vi "Configure Trigger (Glitch).vi"(0 "VISA resource name":refnum<visa-resource-name>, 1 "Maximum Width (1.5E-9s)":dbl=1.5e-09, 5 "Trigger Source (1: Channel 1)":i32(ring)=1 items=["Channel 1"=1, "Channel 2"=2, "Channel 3"=3, "Channel 4"=4, "Digital 0"=13, "Digital 1"=14, "Digital 2"=15, "Digital 3"=16, "Digital 4"=17, "Digital 5"=18, "Digital 6"=19, "Digital 7"=20, "Digital 8"=21, "Digital 9"=22, "Digital 10"=23, "Digital 11"=24, "Digital 12"=25, "Digital 13"=26, "Digital 14"=27, "Digital 15"=28], 7 "Trigger Level (0.0 V)":dbl, 9 "Trigger Polarity (0: Positive)":i32(ring) items=["Positive", "Negative"], 11 "error in (no error)":errorcluster) -> (4 "VISA resource name out":refnum<visa-resource-name>, 15 "error out":errorcluster)   [LabVIEW 2012, in "Agilent 8000 Series.lvlib"]
doc: "Configures the glitch trigger. A glitch trigger occurs when the trigger signal has a pulse with a width that is less than the glitch width. You specify the glitch width in the Glitch Width parameter. You specify the polarity of the pulse with the Glitch Polarity parameter. The trigger does not actually occur until the edge of a pulse that corresponds to the Glitch Width and Glitch Polarity crosses the threshold you specify in the Trigger Level parameter. \n\n<B>Note:</B>\n80000 series oscilloscopes <B>do not</B> support Digital Channels."
uses:
  Agilent 8000 Series.lvlib
panel:
  # "80000 Series Oscilloscopes\ndo not support digital channels"
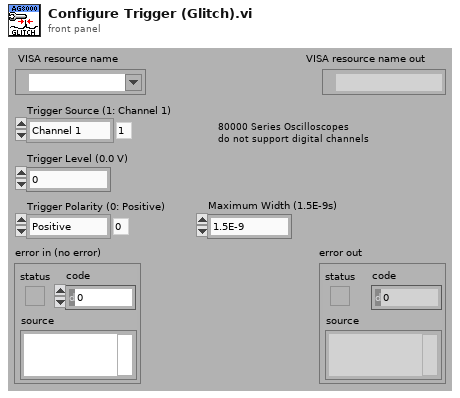
[diagram p1: front panel]
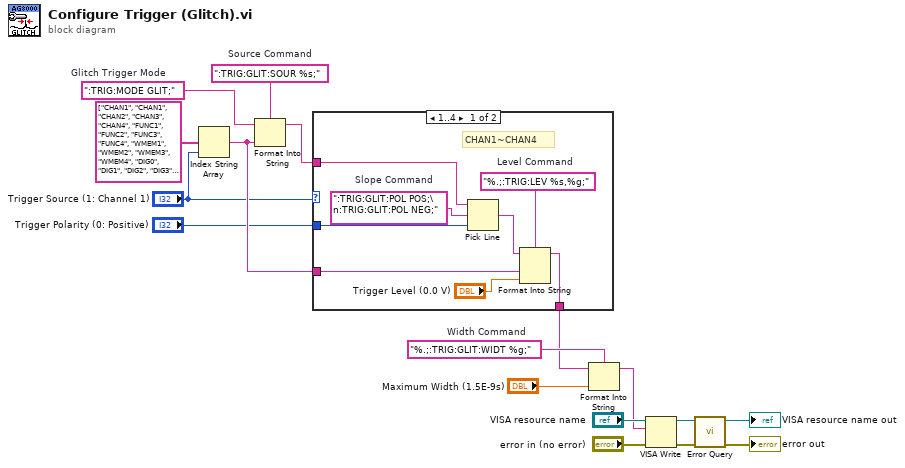
[diagram p0: block diagram]
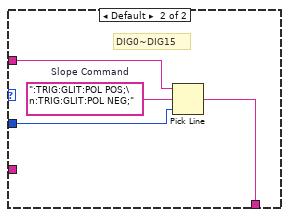
[diagram p2: hidden frame]
diagram:
  w5 = "%.;:TRIG:GLIT:WIDT %g;"  # Width Command
  w10 = ":TRIG:GLIT:SOUR %s;"  # Source Command
  w9 = ":TRIG:MODE GLIT;"  # Glitch Trigger Mode
  n1 = Index String Array(1:"Trigger Source (1: Channel 1)", 2:string[] ["CHAN1", "CHAN1", "CHAN2", "CHAN3", "CHAN4", "FUNC1", "FUNC2", "FUNC3", "FUNC4", "WMEM1", "WMEM2", "WMEM3", "WMEM4", "DIG0", "DIG1", "DIG2", "DIG3", "DIG4", "DIG5", "DIG6", "DIG7", "DIG8", "DIG9", "DIG10", "DIG11", "DIG12", "DIG13", "DIG14", "DIG15", "AUX", "LINE"]) -> (0:w7:string)  [unwired: 1 in]
  n2 = Format Into String(format string=w10, initial string=w9, w7) -> (resulting string=w8:string)  [unwired: 1 in, 1 out]
  n3 = case shown="1..4" "Trigger Source (1: Channel 1)" {
    tunnel: [w24 w26] -> w3
    tunnel: "Trigger Polarity (0: Positive)" -> [w21 w28]
    tunnel: w8 -> [w22 w27]
    tunnel: w7 -> [w19 _]
    frame 1..4 {
      w23 = ":TRIG:GLIT:POL POS;\n:TRIG:GLIT:POL NEG;"  # Slope Command
      w25 = "%.;:TRIG:LEV %s,%g;"  # Level Command
      # "CHAN1~CHAN4"
      n4 = Pick Line(string ("")=w22, multi-line string=w23, line index=w21) -> (output string=w20:string)
      n5 = Format Into String(format string=w25, initial string=w20, w19, "Trigger Level (0.0 V)") -> (resulting string=w24:string)  [unwired: 1 in, 1 out]
    }
    frame Default {
      w29 = ":TRIG:GLIT:POL POS;\n:TRIG:GLIT:POL NEG;"  # Slope Command
      # "DIG0~DIG15"
      n6 = Pick Line(string ("")=w27, multi-line string=w29, line index=w28) -> (output string=w26:string)
    }
  }
  n7 = Format Into String(format string=w5, initial string=w3, "Maximum Width (1.5E-9s)") -> (resulting string=w2:string)  [unwired: 1 in, 1 out]
  n8 = VISA Write(VISA resource name="VISA resource name", write buffer=w2, error in (no error)="error in (no error)") -> (VISA resource name out=w13:refnum<visa-resource-name>, error out=w12:errorcluster)  [unwired: 1 out]
  n9 = call "Error Query.vi"("error in (no error)"=w12, "VISA resource name"=w13) -> ("error out"=→"error out":errorcluster, "VISA resource name out"=→"VISA resource name out":refnum<visa-resource-name>)  [unwired: 6 in, 2 out]
